vi "energyGraph.vi"(8 "error in (no error)":errorcluster, 10 "Clean+No Dups":string[][](array[string]), 11 "CSV Input File":path) -> (0 "error out":errorcluster, 2 "Clean+No Dups Out":string[][](array[string]), 3 "Histogram Graph":T1(graph))   [LabVIEW 2019]
uses:
  <vilib>/Analysis/NI_AALBase.lvlib
panel:
  out "number":u32[](array[numeric])
  out "Energy":string[](array[string])
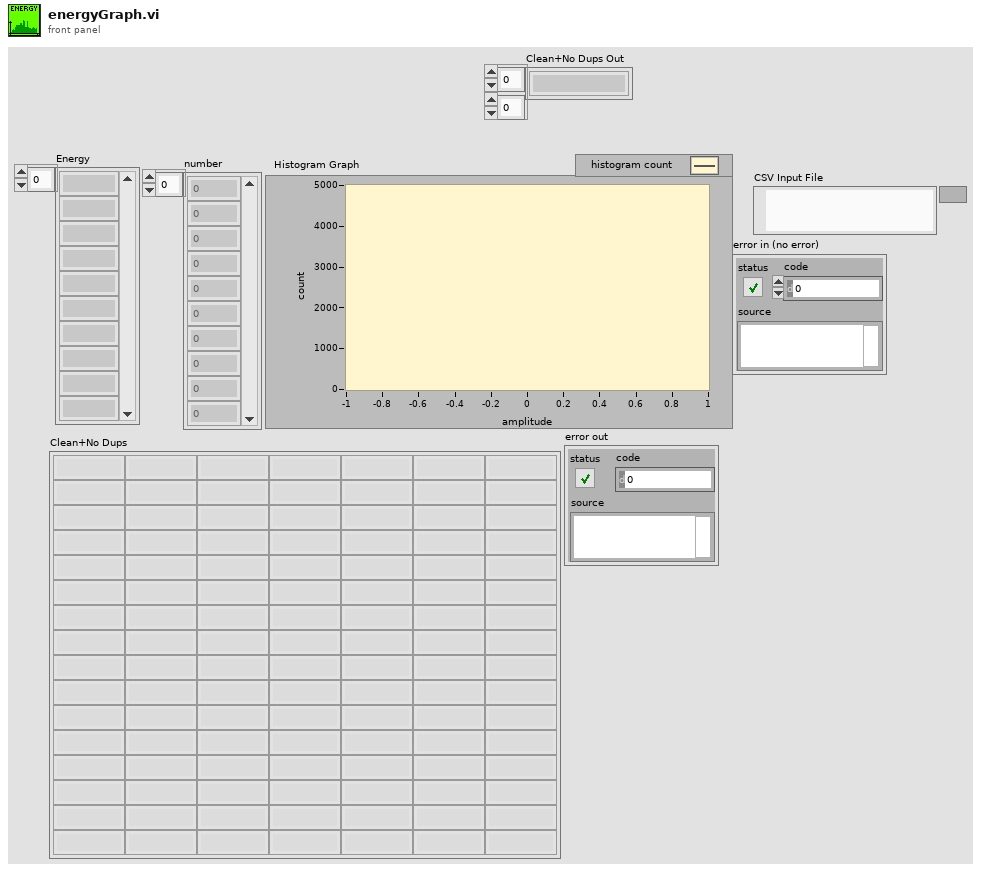
[diagram p1: front panel]
types:
  T1 = cluster{"X Values":dbl[], "Histogram: h(x)":i32[]}
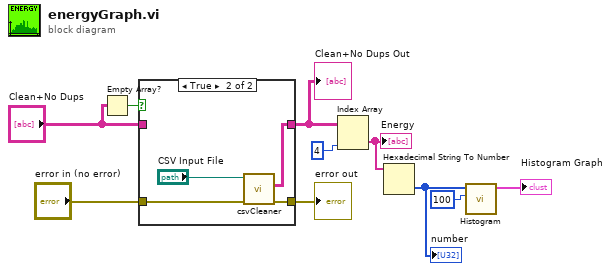
[diagram p0: block diagram]
diagram:
  n1 = Empty Array?(array="Clean+No Dups") -> (empty?=w5:bool)
  n2 = case shown="True" w5 {
    tunnel: [w12 w15] -> w6
    tunnel: "Clean+No Dups" -> [w12 _]
    tunnel: "error in (no error)" -> [w11 w14]
    tunnel: [w11 w13] -> w2
    frame False {
    }
    frame True {
      n3 = call "csvCleaner.vi"("error in (no error)"=w14, "CSV Input File"="CSV Input File") -> ("error out"=w13:errorcluster, "Clean+No Dups"=w15:string[][])  [unwired: 2 in, 6 out]
    }
  }
  "error out" <- w2
  "Clean+No Dups Out" <- w6
  n4 = Index Array(array=w6, index (col)=4 ("disabled index (col)")) -> (element=w9:string[])  [unwired: 1 in]
  "Energy" <- w9
  n5 = Hexadecimal String To Number(string=w9) -> (number=w1:u32[])  [unwired: 2 in, 1 out]
  "number" <- w1
  n6 = call <vilib>:"Histogram.vi"("intervals"=100, "X"=w1) -> ("Histogram Graph"=→"Histogram Graph":T1)  [unwired: 5 in, 4 out]
